vi "应用举例_秒表.vi"() -> ()   [LabVIEW 2013]
panel:
  in  "停止":bool
  out "数码管":dbl(xcontrol)
  # "LED_V1.1  By Bincker @ LabVIEW Fan"
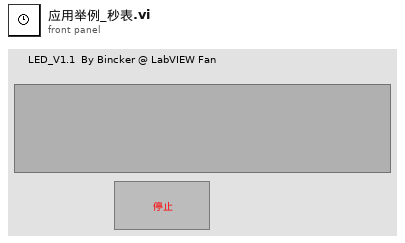
[diagram p1: front panel]
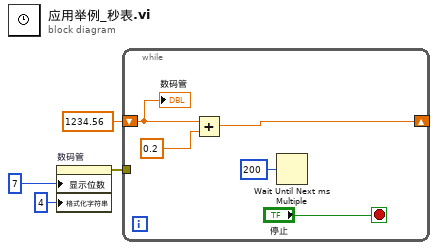
[diagram p0: block diagram]
diagram:
  n1 = property on="数码管" class="数码管 (严格)"("显示位数"=u8 7, "格式化字符串"=u8 4 ("小数位数")) -> (error out=w4:errorcluster)  [unwired: 2 in, 1 out]
  n2 = while {
    tunnel: w4 -> [_]
    shift-right: [w5] -> _
    shift-left: 1234.56 -> [w6]
    stop <- "停止" stop-if-true
    n3 = Add(x=w6, y=0.2) -> (x+y=w5:dbl)
    n4 = Wait Until Next ms Multiple(millisecond multiple=u32 200 ("毫秒倍数")) -> ()  [unwired: 1 out]
    "数码管" <- w6
  }
